vi "AddProject.vi"(8 "error in (no error)":errorcluster, 11 "DB in":refnum<class "DB.lvclass">) -> (0 "error out":errorcluster, 3 "DB out":refnum<class "DB.lvclass">)   [LabVIEW 2015, in "DB.lvclass"]
uses:
  DB.lvclass
  DB.lvclass/DB.ctl
  <vilib>/drjdpowell/SQLite Library/SQL Statement/SQL Statement.lvclass/SQL Statement.ctl
  <vilib>/drjdpowell/SQLite Library/SQL Connection/Open (path).vi
  <vilib>/drjdpowell/SQLite Library/SQL Statement/Bind Text.vi
  <vilib>/drjdpowell/SQLite Library/SQL Connection/Open (string).vi
  <vilib>/drjdpowell/SQLite Library/SQL Statement/Step.vi
  <vilib>/AdvancedString/Path To Command Line String.vi
  <vilib>/drjdpowell/SQLite Library/SQL Statement/Error Message.vi
  <vilib>/drjdpowell/SQLite Library/SQL Connection/Connection.lvclass
  <vilib>/drjdpowell/SQLite Library/SQL Statement/SQL Statement.lvclass
  <vilib>/drjdpowell/SQLite Library/Transaction Helpers/Transaction.lvlib
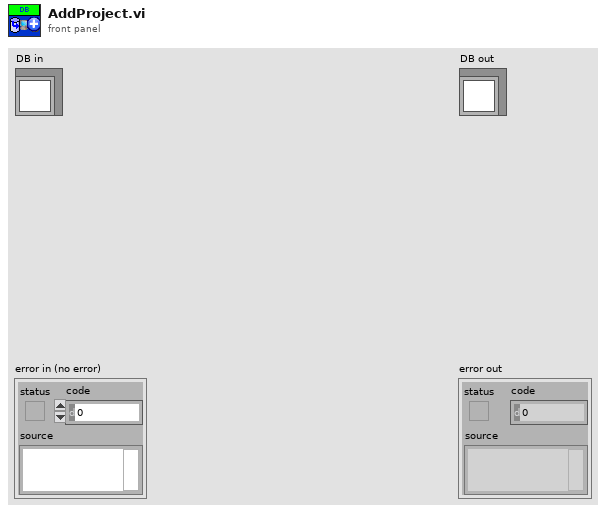
[diagram p1: front panel]
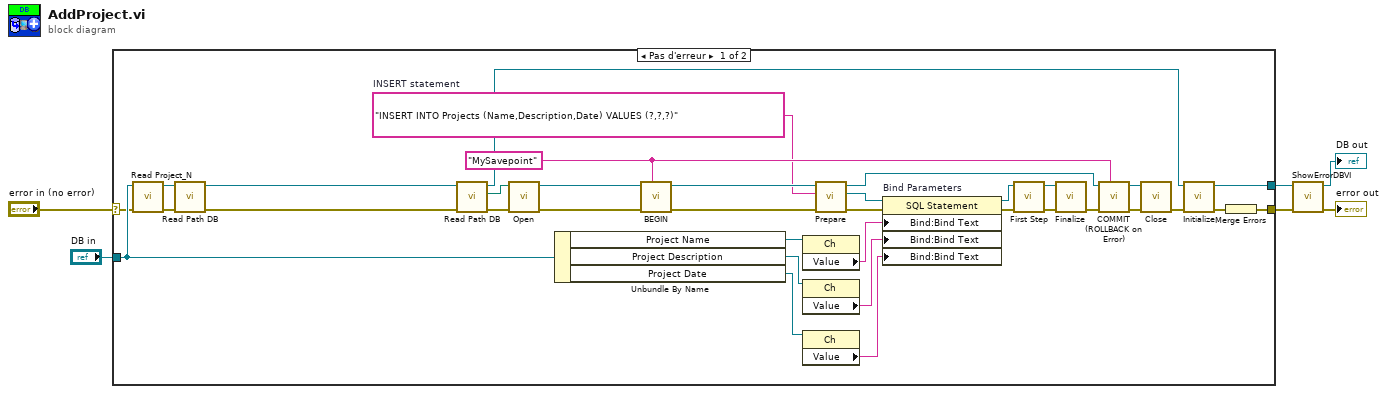
[diagram p0: block diagram]
diagram:
  n1 = case shown="Pas d'erreur" "error in (no error)" {
    selector: "error in (no error)" -> [w29 w43]
    tunnel: [w41 w43] -> w4
    tunnel: [w16 w42] -> w2
    tunnel: "DB in" -> [w31 w42]
    frame No Error {
      w36 = "MySavepoint" ("Savepoint name")
      w7 = "INSERT INTO Projects (Name,Description,Date) VALUES (?,?,?)"  # INSERT statement
      n2 = call "Read Project_N.vi"("error in (no error)"=w29, "DB in"=w31) -> ("error out"=w28:errorcluster, "DB out"=w30:refnum<class "DB.lvclass">)  [unwired: 7 in, 1 out]
      n3 = call "Read Path DB.vi"("error in (no error)"=w28, "DB in"=w30) -> ("error out"=w27:errorcluster, "DB out"=w24:refnum<class "DB.lvclass">)  [unwired: 7 in, 1 out]
      n4 = call "Read Path DB.vi"("error in (no error)"=w27, "DB in"=w24) -> ("error out"=w25:errorcluster, "Path DB"=w26:path, "DB out"=w18:refnum<class "DB.lvclass">)  [unwired: 7 in]
      n5 = call-poly <vilib>:"Open.vi"("error in (no error)"=w25, "db file"=w26) -> ("error out"=w22:errorcluster, "SQLite Connection out"=w23:refnum<class "Connection.lvclass">)  [unwired: 8 in]
      n6 = Unbundle By Name(w31) -> ("Project Name"=w15:refnum<vi>, "Project Description"=w14:refnum<vi>, "Project Date"=w13:refnum<vi>)
      n7 = call <vilib>:"BEGIN.vi"("Savepoint name"=w36, "error in (no error)"=w22, "Connection in"=w23) -> ("error out"=w37:errorcluster, "Connection out"=w38:refnum<class "Connection.lvclass">)  [unwired: 7 in]
      n8 = property class="Ch"(reference=w15) -> ("Value"=w8:string)  [unwired: 1 in, 2 out]
      n9 = property class="Ch"(reference=w14) -> ("Value"=w9:string)  [unwired: 1 in, 2 out]
      n10 = property class="Ch"(reference=w13) -> ("Value"=w10:string)  [unwired: 1 in, 2 out]
      n11 = call <vilib>:"Prepare.vi"("error in (no error)"=w37, "SQL"=w7, "SQLite Connection in"=w38) -> ("error out"=w39:errorcluster, "SQL Statement out"=w40:refnum<class "SQL Statement.lvclass">, "SQLite Connection out"=w35:refnum<class "Connection.lvclass">)  [unwired: 4 in, 2 out]
      n12 = property on="Bind Parameters" class="SQL Statement"(reference=w40, error in=w39, "Bind:Bind Text"=w8, "Bind:Bind Text"=w9, "Bind:Bind Text"=w10) -> (reference out=w33:refnum<class "SQL Statement.lvclass">, error out=w32:errorcluster)
      n13 = call <vilib>:"First Step.vi"("error in (no error)"=w32, "SQL Statement in"=w33) -> ("error out"=w11:errorcluster, "SQL Statement out"=w12:refnum<class "SQL Statement.lvclass">)  [unwired: 7 in, 1 out]
      n14 = call <vilib>:"Finalize.vi"("error in (no error)"=w11, "SQL Statement in"=w12) -> ("error out"=w34:errorcluster)  [unwired: 9 in]
      n15 = call <vilib>:"COMMIT (ROLLBACK on Error).vi"("Savepoint name"=w36, "error in (no error)"=w34, "Connection in"=w35) -> ("error out"=w21:errorcluster, "Connection out"=w20:refnum<class "Connection.lvclass">)  [unwired: 7 in]
      n16 = call-dynamic "Close.vi"("error in (no error)"=w21, "SQLite Connection in"=w20) -> ("error out"=w19:errorcluster)  [unwired: 9 in]
      n17 = call "Initialize.vi"("error in (no error)"=w19, "DB in"=w18) -> ("error out"=w17:errorcluster, "DB out"=w16:refnum<class "DB.lvclass">)  [unwired: 8 in]
      n18 = Merge Errors(w17) -> (w41:errorcluster)
    }
    frame Error {
    }
  }
  n19 = call "ShowErrorDBVI.vi"("error in (no error)"=w4, "DB in"=w2) -> ("error out"=→"error out":errorcluster, "DB out"=→"DB out":refnum<class "DB.lvclass">)  [unwired: 8 in]
